vi "JSON Array.vi"(8 "error in (no error)":errorcluster, 10 "Start Index":i32, 11 "JSON":string) -> (0 "error out":errorcluster, 2 "End Index":i32, 3 "VArray":variant)   [LabVIEW 2011]
panel:
  out "Start Index 2":i32
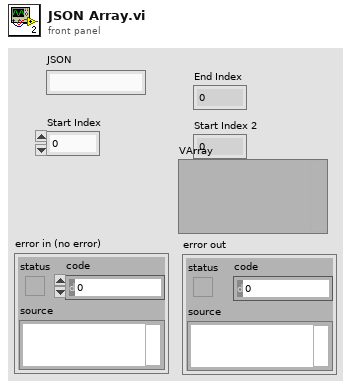
[diagram p1: front panel]
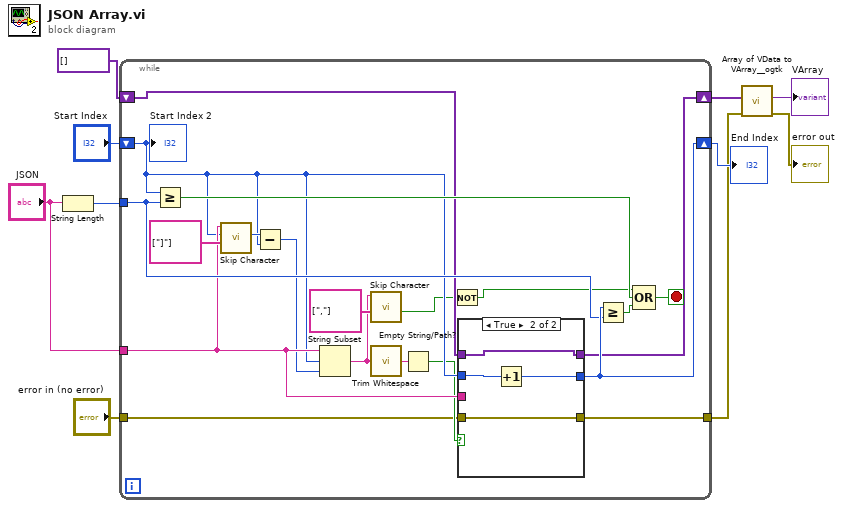
[diagram p0: block diagram]
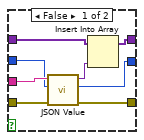
[diagram p2: hidden frame]
diagram:
  n1 = String Length(string="JSON") -> (length=w8:i32)
  n2 = while {
    tunnel: "JSON" -> [w21]
    tunnel: w8 -> [w26]
    shift-right: [w23] -> w5
    shift-left: variant[] [] -> [w24]
    shift-right: [w27] -> w7
    shift-left: "Start Index" -> [w18]
    tunnel: "error in (no error)" -> [w12]
    tunnel: [w11] -> w2
    stop <- w28 stop-if-true
    n3 = Greater Or Equal?(x=w18, y=w26) -> (x >= y?=w29:bool)
    n4 = call "Skip Character.vi"("Stop Strings"=string[] ["]"], "Start Index"=w18, "JSON"=w21) -> ("End Index"=w20:u32)  [unwired: 6 in, 2 out]
    n5 = Subtract(x=w20, y=w18) -> (x-y=w19:u32)
    n6 = String Subset(string=w21, offset (0)=w18, length (rest)=w19) -> (substring=w15:string)
    n7 = call "Skip Character.vi"("Stop Strings"=string[] [","], "JSON"=w15) -> ("Found Stop Character"=w17:bool)  [unwired: 7 in, 2 out]
    n8 = call <vilib>:"Trim Whitespace.vi"("string"=w15) -> ("trimmed string"=w14:string)  [unwired: 1 in]
    n9 = Empty String/Path?(string/path=w14) -> (empty?=w13:bool)
    n10 = Not(x=w17) -> (.not. x?=w16:bool)
    n11 = case shown="True" w13 {
      tunnel: w21 -> [w38 _]
      tunnel: w18 -> [w34 w42]
      tunnel: [w33 w41] -> w27
      tunnel: w24 -> [w37 w40]
      tunnel: [w36 w40] -> w23
      tunnel: w12 -> [w32 w39]
      tunnel: [w31 w39] -> w11
      frame False {
        n12 = call "JSON Value.vi"("error in (no error)"=w32, "Start Index"=w34, "JSON"=w38) -> ("error out"=w31:errorcluster, "End Index"=w33:u32, "Value"=w35:variant)  [unwired: 6 in]
        n13 = Insert Into Array(array=w37, new element=w35) -> (w36:variant[])  [unwired: 1 in]
      }
      frame True {
        n14 = Increment(x=w42) -> (x+1=w41:u32)
      }
    }
    n15 = Greater Or Equal?(x=w27, y=w26) -> (x >= y?=w25:bool)
    n16 = Compound Arithmetic op=OR(w16, w29, w25) -> (w28:bool)
    "Start Index 2" <- w18
  }
  "End Index" <- w7
  n17 = call <userlib>:"Array of VData to VArray__ogtk.vi"("error in (no error)"=w2, "1D Array of VData"=w5) -> ("error out"=→"error out":errorcluster, "VArray"=→"VArray":variant)  [unwired: 8 in]
